vi "Load Config.vi"(8 "error in (no error)":errorcluster, 11 "PluginGUI in":refnum<class "PluginGUI.lvclass">) -> (0 "error out":errorcluster, 3 "PluginGUI out":refnum<class "PluginGUI.lvclass">)   [LabVIEW 2020, in "VolatusGUI.lvlib" / "PluginGUI.lvclass"]
uses:
  PluginGUI.lvclass
  C:/dev/lv20CE/relink/lv-volatus/Volatus/Module/Module.lvclass
  Volatus/Module/Module.lvclass/Module.ctl
  VolatusConfig/VolatusConfigElement/VolatusConfigElement.lvclass/VolatusConfigElement.ctl
  PluginGUI.lvclass/PluginGUI.ctl
  Volatus/Module/Config.vi
  VolatusConfig/VolatusConfigElement/Element.vi
  VolatusConfig/Task/Task.lvclass
  C:/dev/lv20CE/relink/lv-volatus/VolatusConfig/VolatusConfigElement/VolatusConfigElement.lvclass
  Volatus/Module/Module.lvclass
  VolatusConfig/VolatusConfigElement/VolatusConfigElement.lvclass
  lv-cdm/CDM-Config/Config Element/Config Element.lvclass
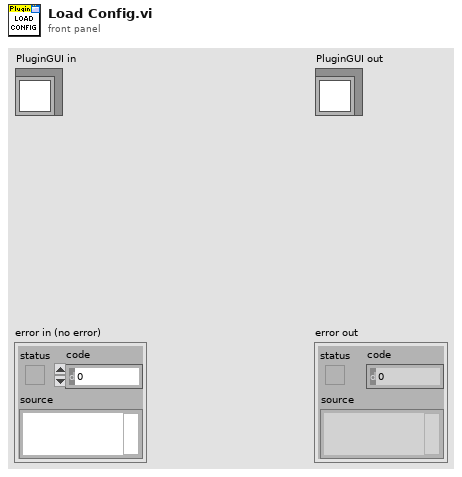
[diagram p1: front panel]
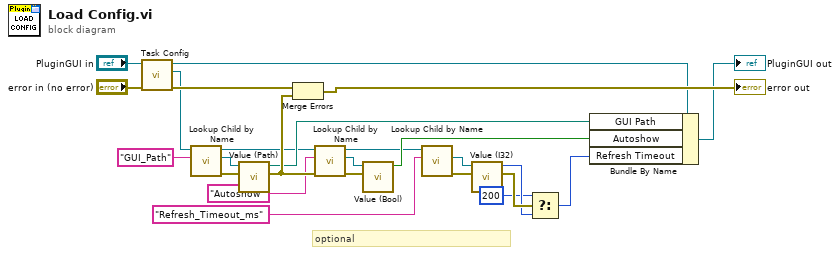
[diagram p0: block diagram]
diagram:
  # "optional"
  n1 = call "Task Config.vi"("error in (no error)"="error in (no error)", "Module in"="PluginGUI in") -> ("error out"=w23:errorcluster, "Task Config"=w21:refnum<class "Task.lvclass">, "Module out"=w10:refnum<class "PluginGUI.lvclass">)  [unwired: 7 in]
  n2 = call "Lookup Child by Name.vi"("Child Name"="GUI_Path", "VolatusConfigElement in"=w21) -> ("error out"=w19:errorcluster, "Child"=w18:refnum<class "Config Element.lvclass">, "VolatusConfigElement out"=w16:refnum<class "Task.lvclass">)  [unwired: 6 in, 1 out]
  n3 = call "Value (Path).vi"("error in (no error)"=w19, "Config Element in"=w18) -> ("error out"=w25:errorcluster, "Path Value"=w17:path)  [unwired: 8 in]
  n4 = Merge Errors(w23, w25) -> (→"error out":errorcluster)
  n5 = call "Lookup Child by Name.vi"("error in (no error)"=w25, "Child Name"="Autoshow", "VolatusConfigElement in"=w16) -> ("error out"=w14:errorcluster, "Child"=w13:refnum<class "Config Element.lvclass">, "VolatusConfigElement out"=w8:refnum<class "Task.lvclass">)  [unwired: 5 in, 1 out]
  n6 = call "Value (Bool).vi"("error in (no error)"=w14, "Config Element in"=w13) -> ("Bool Value"=w12:bool)  [unwired: 8 in, 1 out]
  n7 = call "Lookup Child by Name.vi"("Child Name"="Refresh_Timeout_ms", "VolatusConfigElement in"=w8) -> ("error out"=w6:errorcluster, "Child"=w5:refnum<class "Config Element.lvclass">)  [unwired: 6 in, 2 out]
  n8 = call "Value (I32).vi"("error in (no error)"=w6, "Config Element in"=w5) -> ("error out"=w4:errorcluster, "I32 Value"=w3:i32)  [unwired: 8 in]
  n9 = Select(t=200, s=w4, f=w3) -> (s? t:f=w1:i32)
  n10 = Bundle By Name(cluster=w10, "GUI Path"=w17, "Autoshow"=w12, "Refresh Timeout"=w1) -> (→"PluginGUI out":refnum<class "PluginGUI.lvclass">)
